vi "Main - Process.vi"(8 "error in (no error)":errorcluster) -> (0 "error out":errorcluster)   [LabVIEW 2011]
doc: "This is a basic Queue Driven Message Handler VI. Most advanced LabVIEW programmers who code extensively in LabVIEW utilitze some variation of this VI. This is a starting point. Some key features need to be added. In particular a robust error handling routine should be added.\n\nAAL 9/09"
uses:
  Shared/QDMH Poly VIs/QDMH POLY Enqueue Strings.vi
  Shared/QDMH Poly VIs/QDMH POLY Enqueue String.vi
panel:
  out "Recent Cases":string
  out "Message Display":string
  in  "Cancel":bool
  in  "OK":bool
  # "Run this VI and run Main - Interrupt Process.vi.  When you press the Interrupt Process button, it may interrupt the QDMH in this VI at any time.  That could cause significant errors in the system.  Messages coming in from another source, should be controlled in some manner."
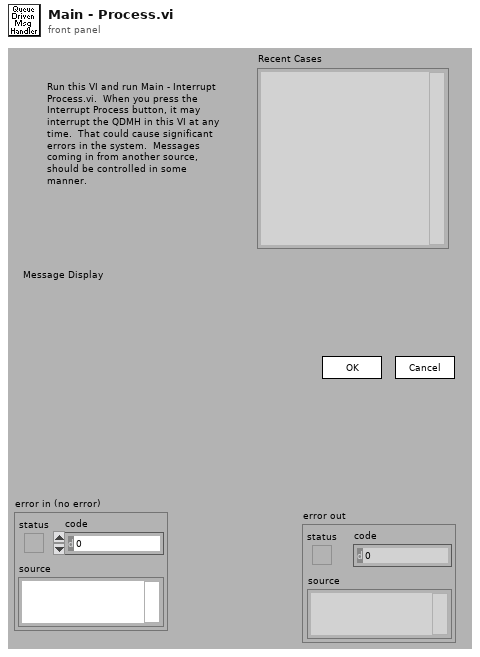
[diagram p1: front panel]
types:
  T1 = cluster{"Operator Name":string, "Current VI's Path":path, "Current VI's  Directory":path, "Queue Names":string[], "# VIs Launched":i32}
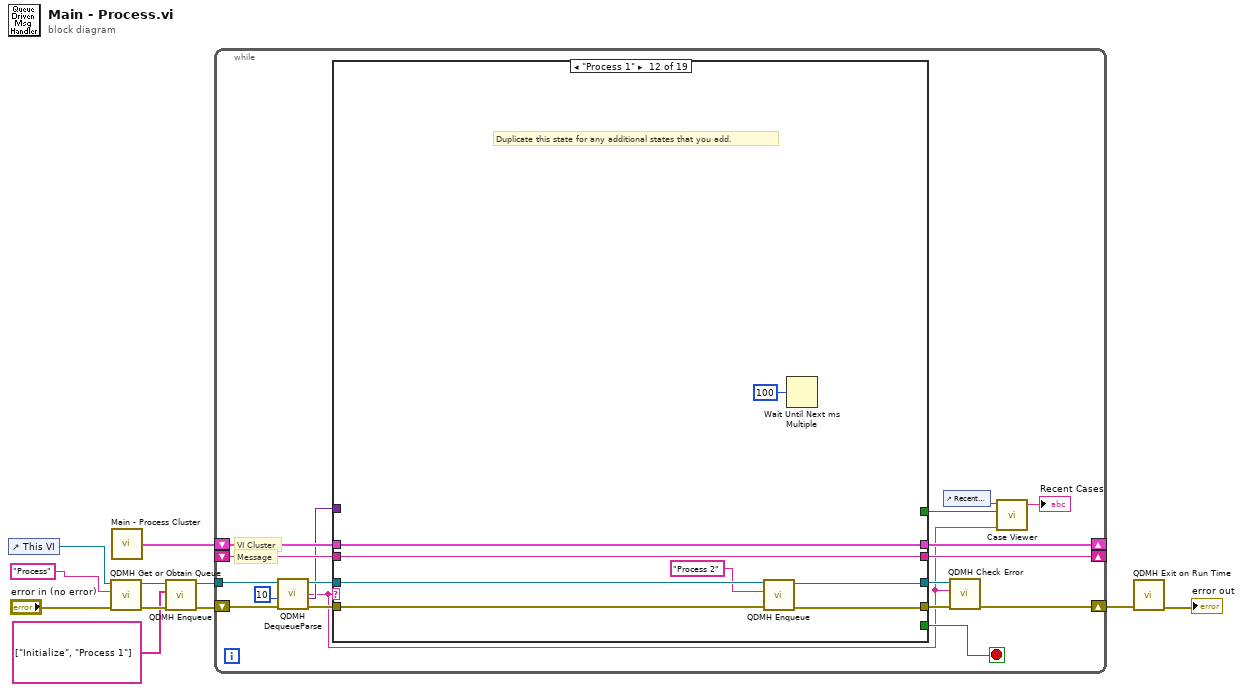
[diagram p0: block diagram]
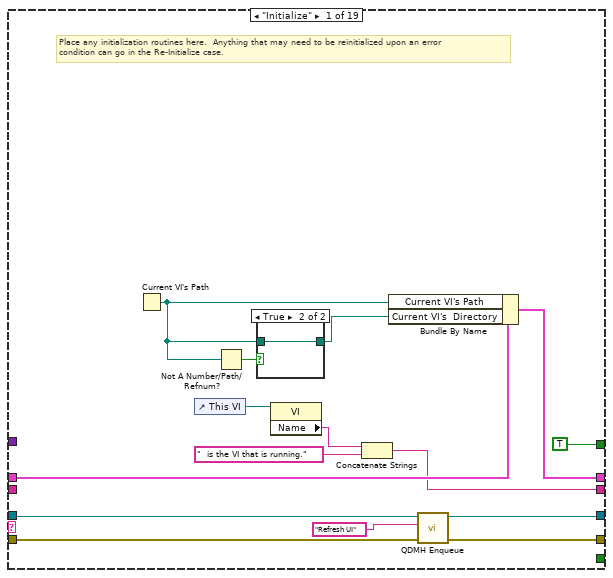
[diagram p2: hidden frame]
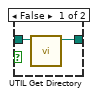
[diagram p3: hidden frame]
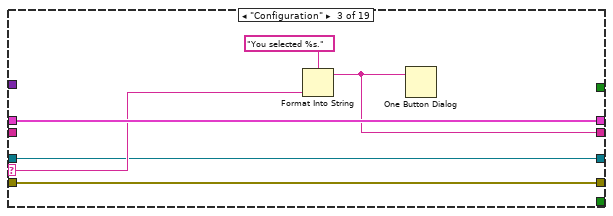
[diagram p5: hidden frame]
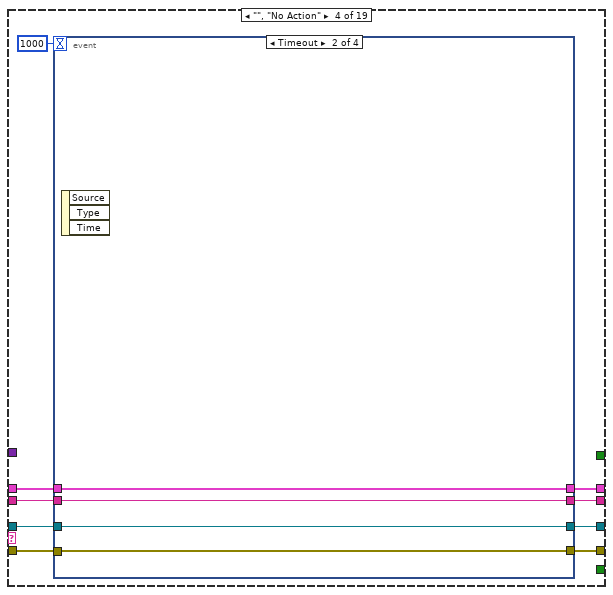
[diagram p6: hidden frame]
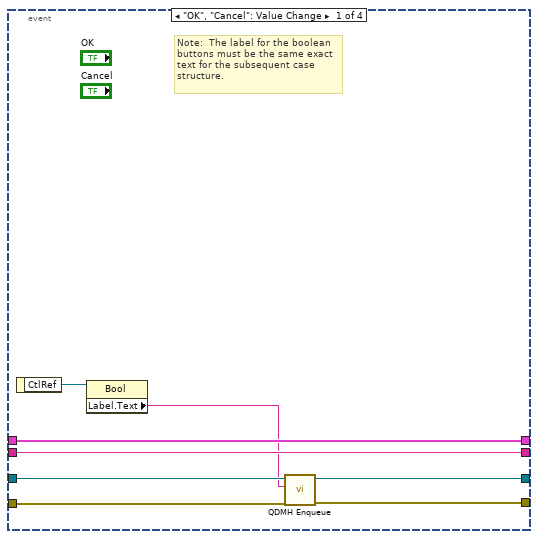
[diagram p7: hidden frame]
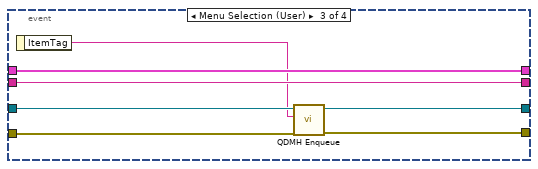
[diagram p8: hidden frame]
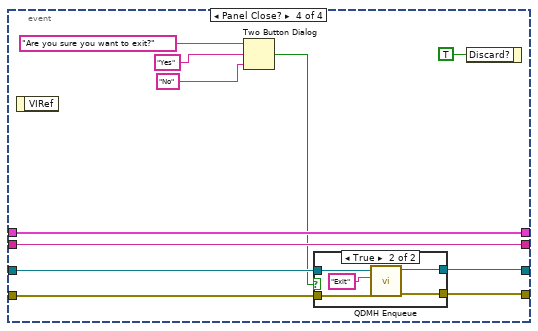
[diagram p9: hidden frame]
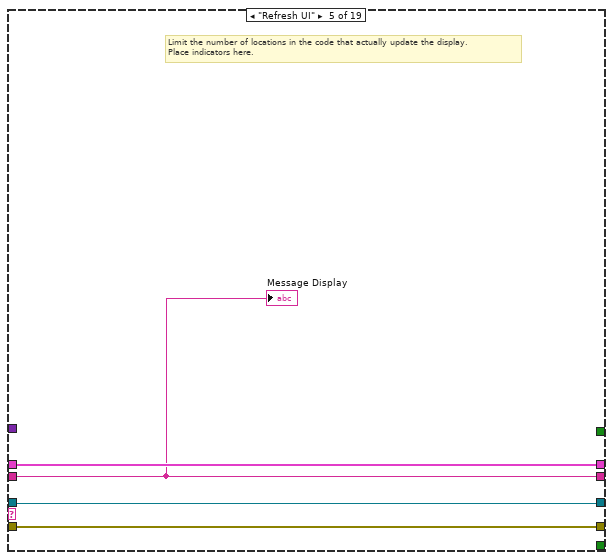
[diagram p11: hidden frame]
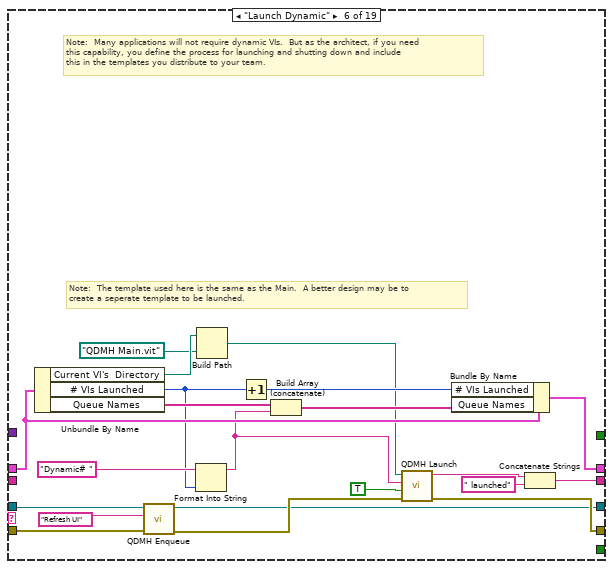
[diagram p12: hidden frame]
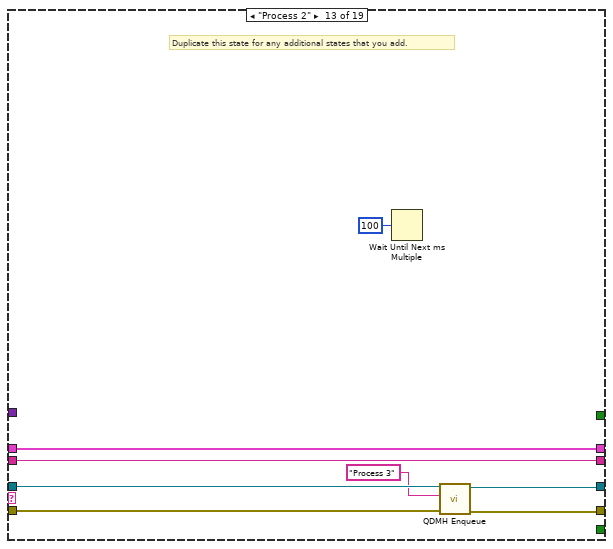
[diagram p18: hidden frame]
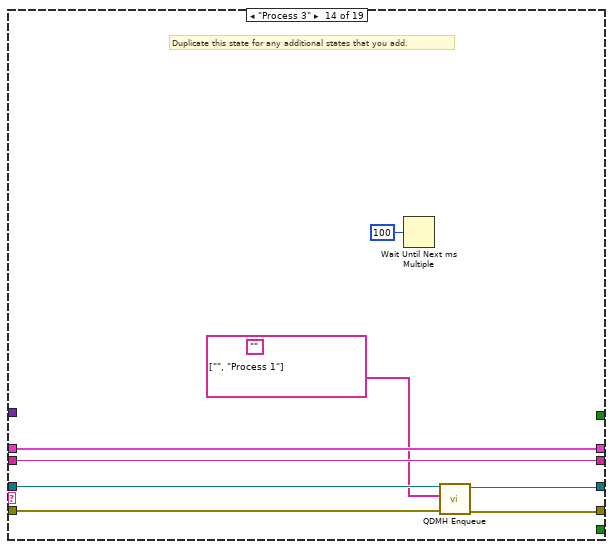
[diagram p19: hidden frame]
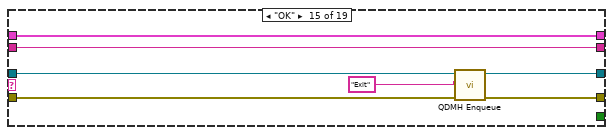
[diagram p20: hidden frame]
diagram:
  n1 = control-ref of="This VI"() -> (w5:refnum<vi>)
  n2 = call "QDMH Get or Obtain Queue.vi"("error in (no error)"="error in (no error)", "Queue Name"="Process", "VI Refnum"=w5) -> ("error out"=w8:errorcluster, "queue out"=w9:refnum<queue>)  [unwired: 7 out]
  n3 = call "Main - Process Cluster.vi"() -> ("Cluster"=w11:T1)
  n4 = call-poly "QDMH Enqueue.vi"("error in (no error)"=w8, "States"=string[] ["Initialize", "Process 1"], "queue"=w9) -> ("error out"=w6:errorcluster, "queue out"=w7:refnum<queue>)  [unwired: 7 out]
  n5 = while {
    tunnel: w7 -> [w24]
    shift-left: w11 -> [w25]
    shift-right: [w26] -> _
    shift-left: _ -> [w27]
    shift-right: [w28] -> _
    shift-right: [w18] -> w4
    shift-left: w6 -> [w20]
    stop <- w29 stop-if-true
    # "VI Cluster"
    # "Message"
    n6 = call "QDMH DequeueParse.vi"("error in (no error)"=w20, "Timeout"=10 ("ms timeout (-1)"), "queue"=w24) -> ("error out"=w21:errorcluster, "Variant Data"=w16:variant, "State"=w12:string, "queue out"=w22:refnum<queue>)  [unwired: 5 out]
    n7 = case shown="\"Process 1\"" w12 {
      selector: w12 -> [_ _ w54 _ _ _ _ _ _ _ _ _ _ _ _ _ _ w199 _]
      tunnel: w22 -> [w40 w48 w53 w66 w105 w124 w129 w133 w137 w141 w145 w154 w162 w170 w179 w181 w193 w196 w209]
      tunnel: [_ _ _ _ _ _ _ _ _ _ _ _ _ _ _ _ _ _ TRUE] -> w29
      tunnel: [w38 w51 w55 w59 w106 w125 w132 w136 w140 w144 w148 w156 w164 w172 w178 w183 w195 w202 w211] -> w28
      tunnel: w27 -> [_ w51 _ w60 w106 _ w132 w136 w140 w144 w148 w156 w164 w172 w178 w183 w195 w202 w211]
      tunnel: [w43 w50 w57 w61 w107 w121 w131 w135 w139 w143 w147 w155 w163 w171 w177 w182 w194 w201 w206] -> w26
      tunnel: w25 -> [w44 w50 w57 w62 w107 w122 w131 w135 w139 w143 w147 w155 w163 w171 w177 w182 w194 w201 w206]
      tunnel: w21 -> [w42 w49 w52 w65 w104 w115 w130 w134 w138 w142 w146 w153 w161 w169 w176 w180 _ w198 w208]
      tunnel: [w41 w49 w52 w64 w104 w114 w130 w134 w138 w142 w146 w151 w159 w167 w175 w180 w192 w198 w203] -> w19
      tunnel: [w33 w48 w53 w58 w105 w111 w129 w133 w137 w141 w145 w152 w160 w168 w173 w181 w191 w196 refnum<queue> refnum ("queue out")] -> w17
      tunnel: w16 -> [_ _ _ _ _ _ _ _ _ _ _ _ _ _ _ _ w189 _ _]
      tunnel: [TRUE _ _ _ _ _ _ _ _ _ _ _ _ _ _ _ _ _ _] -> w14
      frame "Initialize" {
        # "Place any initialization routines here.  Anything that may need to be reinitialized upon an error\ncondition can go in the Re-Initialize case."
        n8 = Current VI's Path() -> (path=w31:path)
        n9 = control-ref of="This VI"() -> (w37:refnum<vi>)
        n10 = Not A Number/Path/Refnum?(number/path/refnum=w31) -> (NaN/Path/Refnum?=w32:bool)
        n11 = case shown="True" w32 {
          tunnel: w31 -> [w46 w47]
          tunnel: [w45 w47] -> w35
          frame False {
            n12 = call "UTIL Get Directory.vi"("Path In"=w46) -> ("Directory Out"=w45:path)  [unwired: 1 in, 9 out]
          }
          frame True {
          }
        }
        n13 = property class="VI"(reference=w37) -> ("Name"=w36:string)  [unwired: 1 in, 2 out]
        n14 = Concatenate Strings(w36, "  is the VI that is running." ("string")) -> (w38:string)
        n15 = Bundle By Name(cluster=w44, "Current VI's Path"=w31, "Current VI's  Directory"=w35) -> (w43:T1)
        n16 = call-poly "QDMH Enqueue.vi"("error in (no error)"=w42, "State"="Refresh UI" ("New State"), "queue"=w40) -> ("error out"=w41:errorcluster, "queue out"=w33:refnum<queue>)  [unwired: 7 out]
      }
      frame "Re-Initialize" {
        # "This case includes initialization functionality that may need to run again during the course of the VI"
      }
      frame "Configuration" {
        n17 = Format Into String(format string="You selected %s." ("Format String"), w54) -> (resulting string=w55:string)  [unwired: 2 in, 1 out]
        n18 = One Button Dialog(message=w55) -> ()  [unwired: 2 out]
      }
      frame "", "No Action" {
        n19 = event shown="[1] Timeout" {
          selector: _ -> [_ _ _ _]
          dyn-events: _ -> [_ _ _ _]
          timeout: 1000 -> [_ _ _ _]
          tunnel: w66 -> [w73 w76 w85 w92]
          tunnel: [w72 w75 w83 w89] -> w64
          tunnel: w65 -> [w71 w75 w84 w91]
          tunnel: w62 -> [w70 w78 w82 w96]
          tunnel: [w70 w78 w82 w96] -> w61
          tunnel: w60 -> [w69 w77 w81 w95]
          tunnel: [w69 w77 w81 w95] -> w59
          tunnel: [w67 w76 w79 w90] -> w58
          event "OK", "Cancel": Value Change {
            # "Note:  The label for the boolean buttons must be the same exact text for the subsequent case structure."
            n20 = event-data() -> ("CtlRef"=w74:refnum<vi>)  [unwired: 1 out]
            n21 = property class="Bool"(reference=w74) -> ("Label.Text"=w68:string)  [unwired: 1 in, 2 out]
            n22 = call-poly "QDMH Enqueue.vi"("error in (no error)"=w71, "State"=w68, "queue"=w73) -> ("error out"=w72:errorcluster, "queue out"=w67:refnum<queue>)  [unwired: 7 out]
          }
          event Timeout {
            n23 = event-data() -> ()  [unwired: 4 out]
          }
          event Menu Selection (User) {
            n24 = event-data() -> ("ItemTag"=w80:string)  [unwired: 1 out]
            n25 = call-poly "QDMH Enqueue.vi"("error in (no error)"=w84, "State"=w80, "queue"=w85) -> ("error out"=w83:errorcluster, "queue out"=w79:refnum<queue>)  [unwired: 7 out]
          }
          event Panel Close? {
            n26 = event-data() -> ()  [unwired: 2 out]
            n27 = Two Button Dialog(message="Are you sure you want to exit?", 1:"No" ("T button name (\"OK\")"), 2:"Yes" ("F button name (\"Cancel\")")) -> (T button?=w86:bool)
            n28 = case shown="True" w86 {
              tunnel: w92 -> [w98 w103]
              tunnel: w91 -> [w97 w102]
              tunnel: [w98 w101] -> w90
              tunnel: [w97 w100] -> w89
              frame False {
              }
              frame True {
                n29 = call-poly "QDMH Enqueue.vi"("error in (no error)"=w102, "State"="Exit", "queue"=w103) -> ("error out"=w100:errorcluster, "queue out"=w101:refnum<queue>)  [unwired: 7 out]
              }
            }
            n30 = event-data("Discard?"=TRUE) -> ()  [unwired: 1 in, 1 out]
          }
        }
      }
      frame "Refresh UI" {
        # "Limit the number of locations in the code that actually update the display.\nPlace indicators here."
        "Message Display" <- w106
      }
      frame "Launch Dynamic" {
        # "Note:  The template used here is the same as the Main.  A better design may be to\ncreate a seperate template to be launched."
        # "Note:  Many applications will not require dynamic VIs.  But as the architect, if you need\nthis capability, you define the process for launching and shutting down and include\nthis in the templates you distribute to your team."
        n31 = Unbundle By Name(w122) -> ("Current VI's  Directory"=w110:path, "# VIs Launched"=w118:i32, "Queue Names"=w120:string[])
        n32 = call-poly "QDMH Enqueue.vi"("error in (no error)"=w115, "State"="Refresh UI" ("New State"), "queue"=w124) -> ("error out"=w113:errorcluster, "queue out"=w111:refnum<queue>)  [unwired: 7 out]
        n33 = Format Into String(initial string="Dynamic# ", w118) -> (resulting string=w116:string)  [unwired: 2 in, 1 out]
        n34 = Build Path(base path=w110, name or relative path=path "QDMH Main.vit" ("vi path")) -> (appended path=w108:path)
        n35 = Increment(x=w118) -> (x+1=w117:i32)
        n36 = Build Array (concatenate)(w120, w116) -> (w119:string[])
        n37 = call "QDMH Launch.vi"("error in (no error)"=w113, "Front Panel Window (Open)"=TRUE ("Front Panel Window:Open"), "Queue Name"=w116, "VI Path"=w108) -> ("error out"=w114:errorcluster, "Launched VI Name"=w127:string)  [unwired: 6 out]
        n38 = Bundle By Name(cluster=w122, "# VIs Launched"=w117, "Queue Names"=w119) -> (w121:T1)
        n39 = Concatenate Strings(w127, " launched" ("string")) -> (w125:string)
      }
      frame "Shutdown Dynamic" {
      }
      frame "Send Message to Dynamic" {
      }
      frame "Receive Message From Dynamic" {
      }
      frame "<duplicate me for new states >" {
        # "Duplicate this state for any additional states that you add."
      }
      frame "Interrupt Process" {
        # "Duplicate this state for any additional states that you add."
      }
      frame "Process 1" {
        # "Duplicate this state for any additional states that you add."
        n40 = call-poly "QDMH Enqueue.vi"("error in (no error)"=w153, "State"="Process 2", "queue"=w154) -> ("error out"=w151:errorcluster, "queue out"=w152:refnum<queue>)  [unwired: 7 out]
        n41 = Wait Until Next ms Multiple(millisecond multiple=u32 100) -> ()  [unwired: 1 out]
      }
      frame "Process 2" {
        # "Duplicate this state for any additional states that you add."
        n42 = Wait Until Next ms Multiple(millisecond multiple=u32 100) -> ()  [unwired: 1 out]
        n43 = call-poly "QDMH Enqueue.vi"("error in (no error)"=w161, "State"="Process 3", "queue"=w162) -> ("error out"=w159:errorcluster, "queue out"=w160:refnum<queue>)  [unwired: 7 out]
      }
      frame "Process 3" {
        (unwired) ""
        # "Duplicate this state for any additional states that you add."
        n44 = Wait Until Next ms Multiple(millisecond multiple=u32 100) -> ()  [unwired: 1 out]
        n45 = call-poly "QDMH Enqueue.vi"("error in (no error)"=w169, "States"=string[] ["", "Process 1"], "queue"=w170) -> ("error out"=w167:errorcluster, "queue out"=w168:refnum<queue>)  [unwired: 7 out]
      }
      frame "OK" {
        n46 = call-poly "QDMH Enqueue.vi"("error in (no error)"=w176, "State"="Exit" ("New State"), "queue"=w179) -> ("error out"=w175:errorcluster, "queue out"=w173:refnum<queue>)  [unwired: 7 out]
      }
      frame "Cancel" {
      }
      frame "Error" {
        # "This codes simply displays an error dialog that will allow the user\nto continue code execution or Exit.  More error correction code\ncould be included.  This will be explored in the error system exercise."
        n47 = Variant To Data(type=cluster{"Case":string, "error":errorcluster} {"Case"="", "error"={"status"=FALSE, "code"=0, "source"=""}} ("QDSM Element"), Variant=w189) -> (data=w188:cluster{"Case":string, "error":errorcluster})  [unwired: 1 in, 1 out]
        n48 = Unbundle By Name(w188) -> ("Case"=w187:string, "error"=w186:errorcluster)
        n49 = call "QDMH Error Dialog.vi"("error"=w186, "Case Error Occured"=w187) -> ("error out (no error)"=w184:errorcluster, "Case to Execute"=w185:string)  [unwired: 8 out]
        n50 = call-poly "QDMH Enqueue.vi"("error in (no error)"=w184, "State"=w185, "queue"=w193) -> ("error out"=w192:errorcluster, "queue out"=w191:refnum<queue>)  [unwired: 7 out]
      }
      frame "Developer Error", Default {
        # "Many eschew the use of string based state machines because of the propensity for\ntypos, prefering instead to use enums.  This case eliminates that concern.\nPerhaps modify to exit the VI."
        n51 = Format Into String(format string="Developer Error (hey dude - typo): The requested state \"%s\" does not exist." ("message"), w199) -> (resulting string=w197:string)  [unwired: 2 in, 1 out]
        n52 = One Button Dialog(message=w197) -> ()  [unwired: 2 out]
      }
      frame "Exit" {
        # "Note:  The release queue function has the force destroy option set to true."
        # "Place any critical clean up routines here."
        n53 = Unbundle By Name(w206) -> ("Queue Names"=w204:string[])
        n54 = Release Queue(queue=w209, force destroy? (F)=TRUE, error in (no error)=w208) -> (error out=w203:errorcluster)  [unwired: 2 out]
        n55 = for {
          tunnel: w204 -> [w216] mode=indexing
          n56 = Obtain Queue(name (unnamed)=w216, element data type=cluster{"State":string, "Variant Data":variant} {"State"="", "Variant Data"=variant} ("QDSM Element")) -> (queue out=w215:refnum<queue>)  [unwired: 3 in, 2 out]
          n57 = call-poly "QDMH Enqueue.vi"("State"="Exit" ("element"), "queue"=w215) -> ()  [unwired: 1 in, 9 out]
        }
        n58 = local write "Message Display"("") -> ()
      }
    }
    n59 = control-ref of="Recent Cases"() -> (w13:refnum<vi>)
    n60 = call "QDMH Check Error.vi"("error in (no error)"=w19, "Case"=w12, "queue"=w17) -> ("error out"=w18:errorcluster)  [unwired: 1 in, 7 out]
    n61 = call "Case Viewer.vi"("Case"=w12, "Flush?"=w14, "Str Refnum"=w13) -> ("Recent Cases"=→"Recent Cases":string)  [unwired: 8 in]
  }
  n62 = call "QDMH Exit on Run Time.vi"("error in (no error)"=w4) -> ("error out"=→"error out":errorcluster)  [unwired: 10 in]
